vi "state machine 2.vi"() -> ()   [LabVIEW 2017]
uses:
  <vilib>/Platform/TimedLoop/XDataNode/timing_clust.ctl
  <vilib>/Platform/TimedLoop/XDataNode/nitl_modes.ctl
  <vilib>/Platform/TimedLoop/XDataNode/wakeup.ctl
  <vilib>/rvi/Emulation/niFpgaGetClockAttributes.vi
  <vilib>/rvi/Emulation/niFpgaSctlEmulationGetInTimedLoop.vi
  <vilib>/rvi/Emulation/niFpgaEmulationReportErrorSimple.vi
  <vilib>/rvi/Emulation/niFpgaProcessEmulError.vi
  <vilib>/rvi/Emulation/niFpgaCriticalErrorInLSC.vi
  <vilib>/rvi/interface/RandomDataEmulation/niFpgaRandomDataHandleErrors.vi
  <vilib>/rvi/eio/common/nirviEmuTemplateMethod_errors.vi
  <vilib>/Platform/TimedLoop/XDataNode/XDataNode.xnode
  <vilib>/rvi/DataTransferAndStorage/Container/XNode/niFpgaContainer.xnode
  <vilib>/rvi/interface/RandomDataEmulation/nirviRandomDataFpgaReadWriteTemplate.vi
  <vilib>/eio/EIONode/EIONode.xnode
  <vilib>/Platform/TimedLoop/XDataNode/XDNodeRunTimeDep.lvlib
panel:
  out "real-time port D monitor":bool[](array[boolean])
  out "real-time port C monitor":bool[](array[boolean])
  out "real-time port B monitor":bool[](array[boolean])
  out "real-time port A monitor":bool[](array[boolean])
  in  "stop":bool
  out "reset LED":bool
  out "run LED":bool
  in  "Reset":bool
  out "load LED":bool
  out "idle LED":bool
  in  "Run":bool
  in  "Load":bool
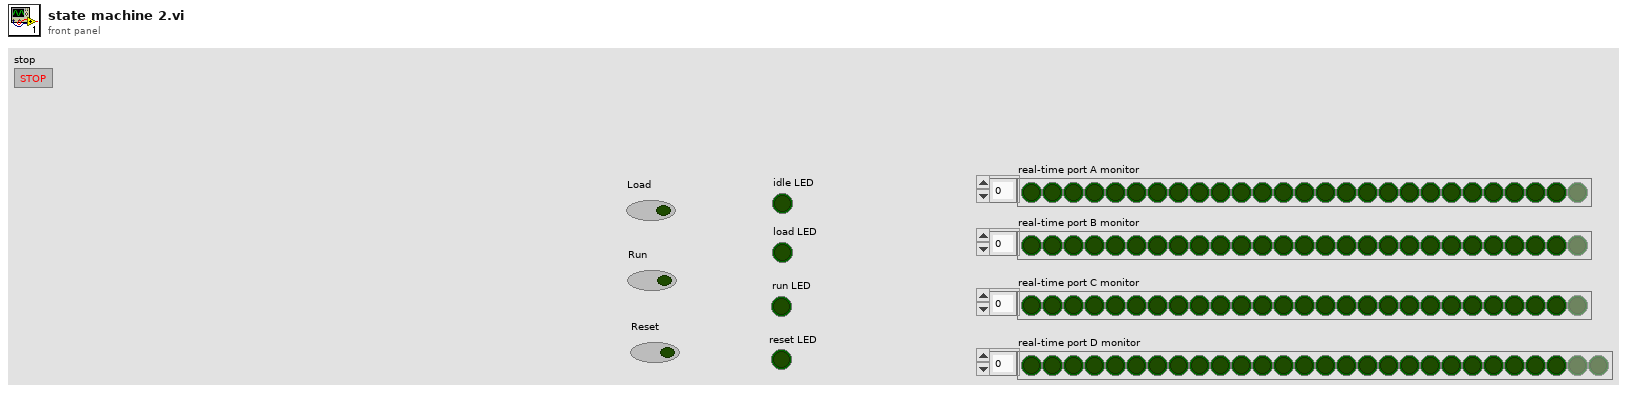
[diagram p1: front panel]
types:
  T1 = typedef "XDNodeRunTimeDep.lvlib/timing_clust.ctl" = cluster{"Expected End [f-1]":u64, "Actual End [f-1]":u64, "Finished Late? [f-1]":bool, "Expected End [i-1]":u64, "Actual End [i-1]":u64, "Finished Late? [i-1]":bool, "Expected Start [i]":u64, "Actual Start [i]":u64, "Expected Start [f]":u64, "Actual Start [f]":u64, "Source Name":string, "Structure Name":string, "Period":i64, "Deadline":i64, "Offset":i64, "Start":i64, "Priority":i32, "Timeout":i32, "Mode":T2, "Wakeup Reason":T3, "Error":errorcluster, "Source Type":string, "Secondary Source Type":string, "Global End Time":u64, "Global Start Time":u64, "Frame Duration":u64, "Iteration Duration":u64, "Assigned CPU":i32, "I/O Scan Engine Mode":u32}
  T2 = typedef "XDNodeRunTimeDep.lvlib/nitl_modes.ctl" = enum32{"No Change", "Process missed periods, maintain original phase", "Discard missed periods, maintain original phase", "Process missed periods, ignore original phase", "Discard missed periods, ignore original phase"}
  T3 = typedef "XDNodeRunTimeDep.lvlib/wakeup.ctl" = enum32{"Normal", "Aborted", "Asynchronous wakeup", "Timing source error", "Timed loop error", "Timeout"}
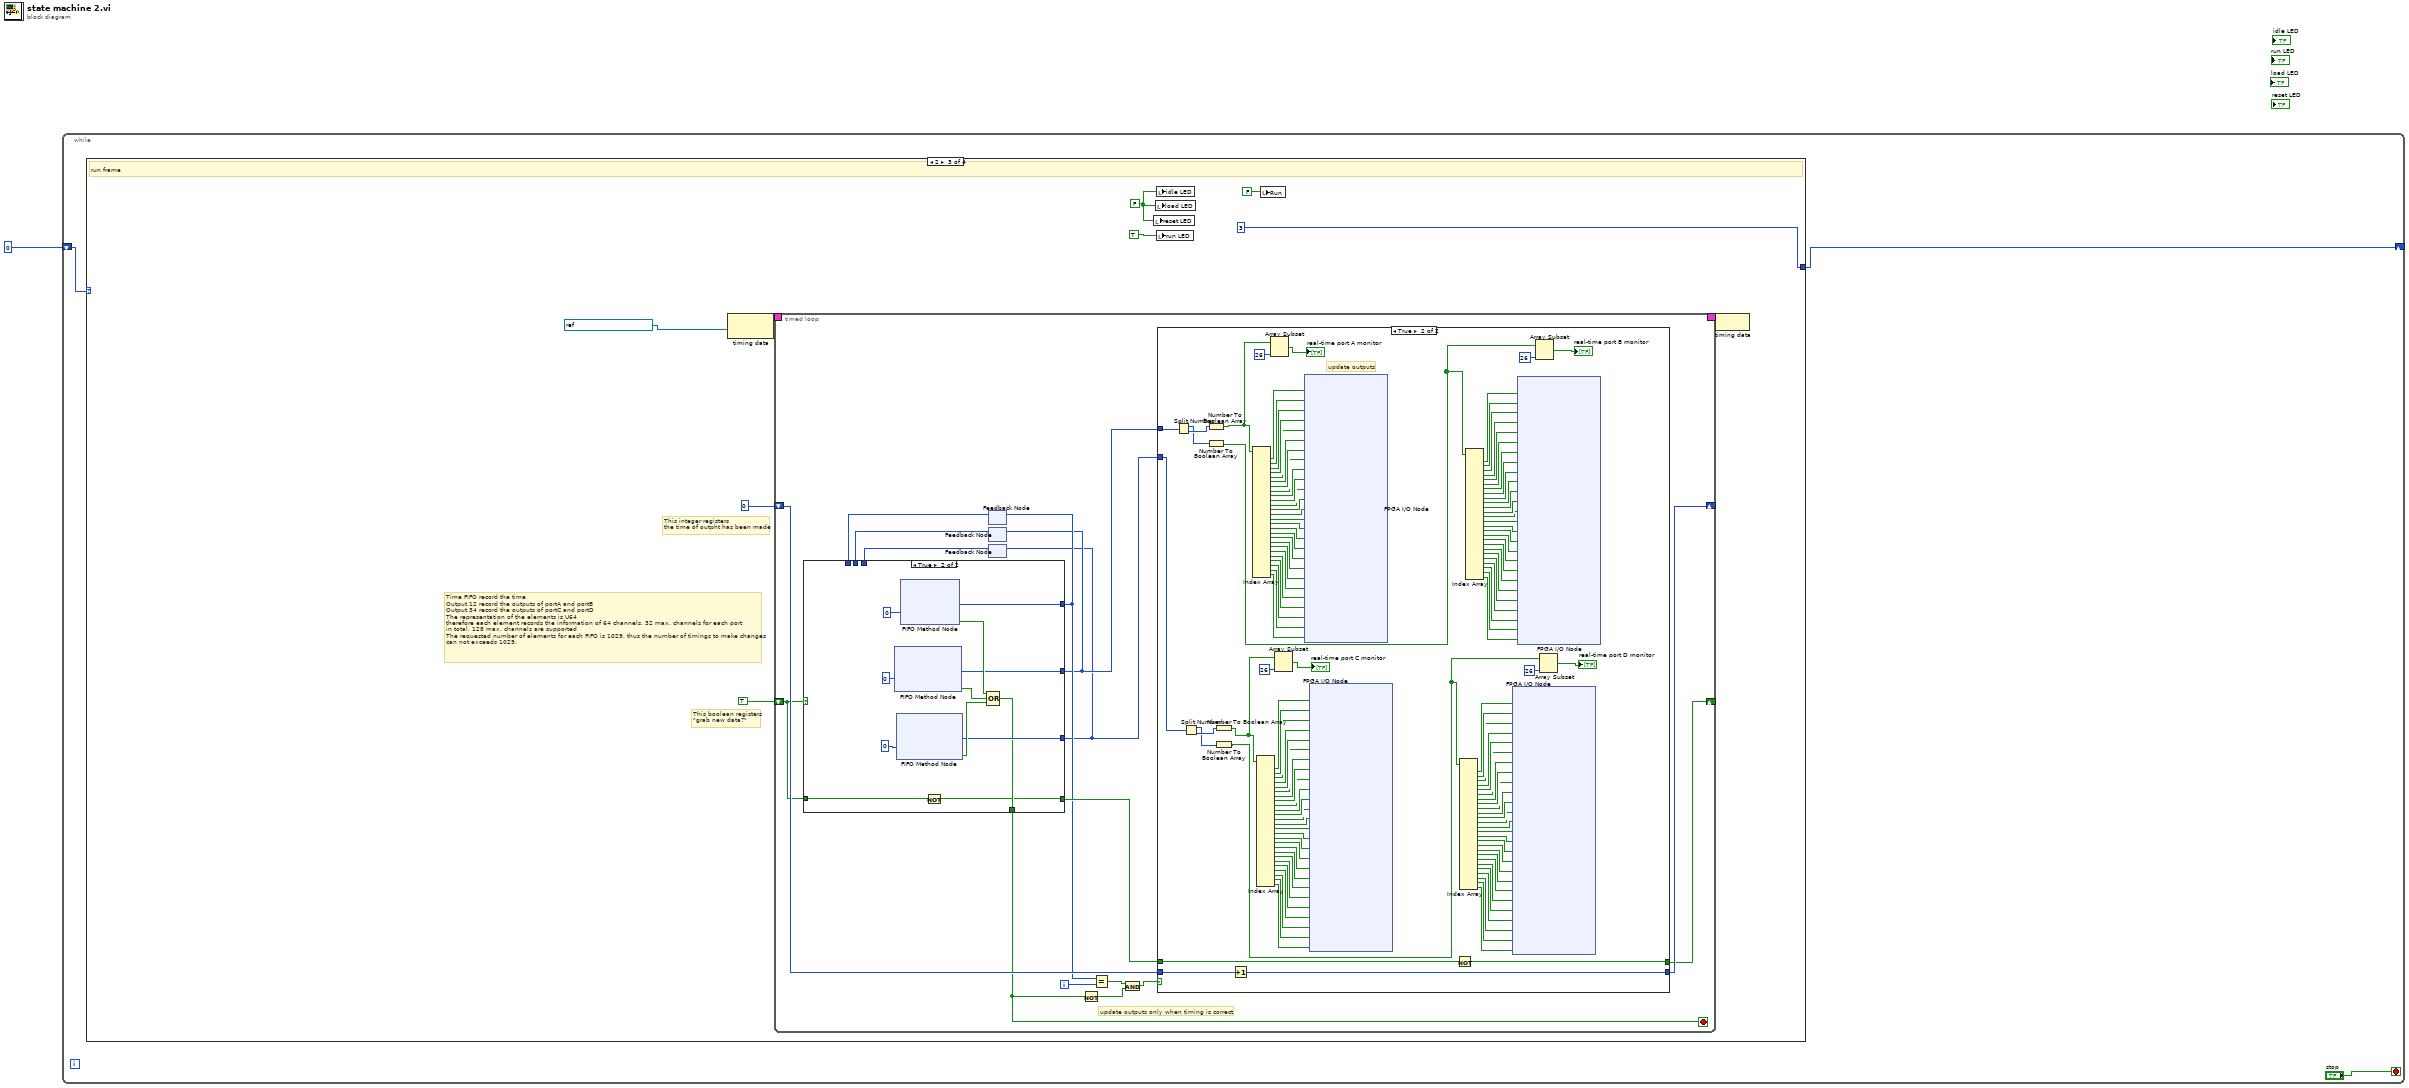
[diagram p0: block diagram]
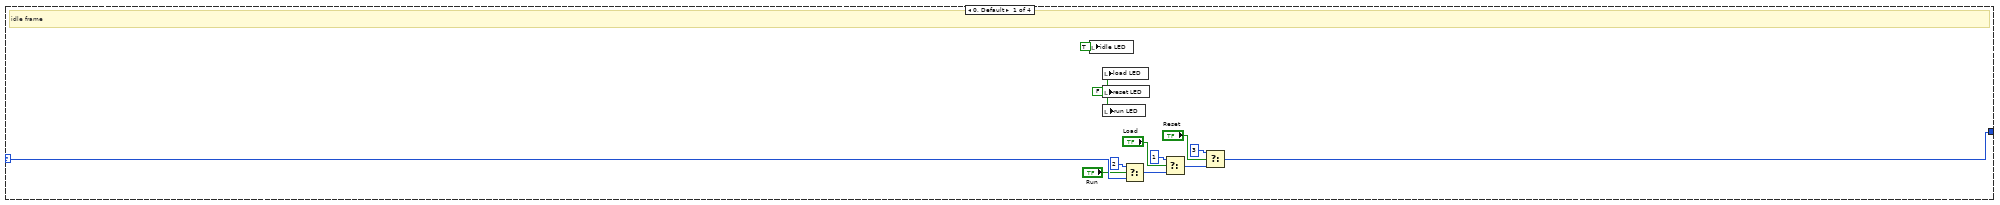
[diagram p2: hidden frame]
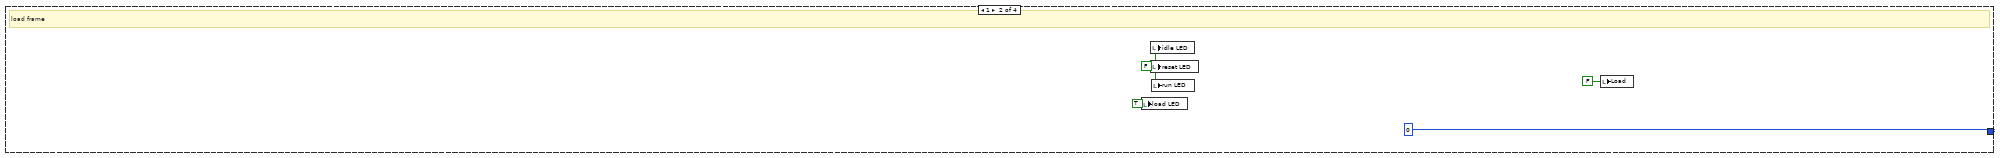
[diagram p3: hidden frame]
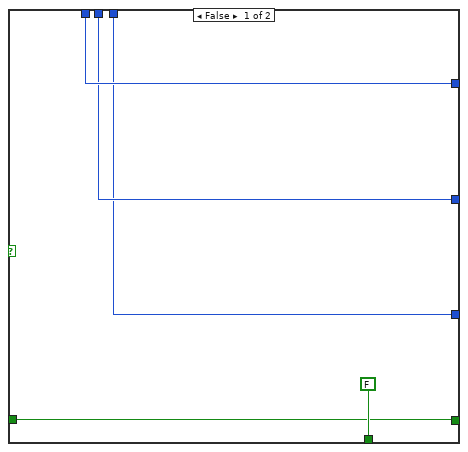
[diagram p4: hidden frame]
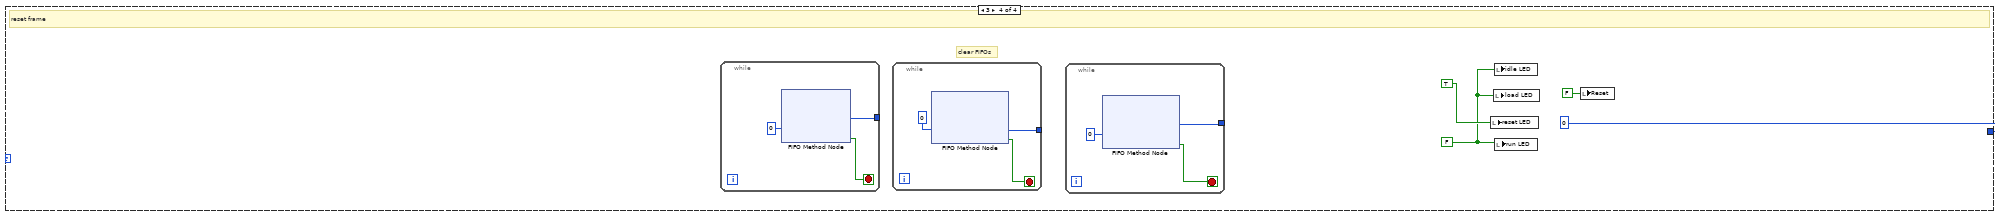
[diagram p6: hidden frame]
diagram:
  n1 = while {
    shift-right: [w3] -> _
    shift-left: i16 0 -> [w4]
    stop <- "stop" stop-if-true
    n2 = case shown="2" w4 {
      selector: w4 -> [w14 _ _ _]
      tunnel: [w7 i16 0 i16 3 i16 0] -> w3
      frame 0, Default {
        w15 = FALSE ("run")
        # "idle frame"
        n3 = local write "idle LED"(TRUE ("run")) -> ()
        n4 = local write "load LED"(w15) -> ()
        n5 = local write "reset LED"(w15) -> ()
        n6 = local write "run LED"(w15) -> ()
        n7 = Select(t=i16 2, s="Run", f=w14) -> (s? t:f=w11:i16)
        n8 = Select(t=i16 1, s="Load", f=w11) -> (s? t:f=w9:i16)
        n9 = Select(t=i16 3, s="Reset", f=w9) -> (s? t:f=w7:i16)
      }
      frame 1 {
        w20 = FALSE ("run")
        # "load frame"
        n10 = local write "load LED"(TRUE ("load")) -> ()
        n11 = local write "idle LED"(w20) -> ()
        n12 = local write "reset LED"(w20) -> ()
        n13 = local write "run LED"(w20) -> ()
        n14 = local write "Load"(FALSE) -> ()
      }
      frame 2 {
        w28 = FALSE ("run")
        # "This integer registers \nthe time of outpht has been made"
        # "This boolean registers\n\"grab new data?\""
        # "Time FIFO record the time\nOutput 12 record the outputs of portA and portB\nOutput 34 record the outputs of portC and portD\nThe representation of the elements is U64\ntherefore each element records the information of 64 channels, 32 max. channels for each port\nin total, 128 max. channels are supported\nThe requested number of elements for each FIFO is 1029, thus the number of timings to make changes \ncan not exceeds 1029."
        # "run frame"
        n15 = node-c288(refnum<k21> "40 MHz Onboard Clock" ("Source Name")) -> (w26:T1)
        n16 = timed-loop {
          timing: w26 -> [_]
          timing-out: [_] -> w25
          shift-right: [w43] -> _
          shift-left: i16 0 -> [w44]
          shift-right: [w37] -> _
          shift-left: TRUE ("Boolean") -> [w36]
          i -> [w45]
          stop <- w40 stop-if-true
          # "update outputs only when timing is correct"
          n17 = feedback #1() -> (w32:u64)  [unwired: 1 in]
          n18 = feedback #2() -> (w31:u64)  [unwired: 1 in]
          n19 = feedback #3() -> (w30:u64)  [unwired: 1 in]
          n20 = case shown="True" w36 {
            tunnel: [w47 w56] -> w34
            tunnel: [w46 w55] -> w33
            tunnel: [w48 w54] -> w35
            tunnel: [FALSE w53] -> w40
            tunnel: w36 -> [w49 w52]
            tunnel: [w49 w51] -> w38
            tunnel: w32 -> [w48 _]
            tunnel: w31 -> [w47 _]
            tunnel: w30 -> [w46 _]
            frame False {
            }
            frame True {
              n21 = xnode ("FIFO Method Node")("Timeout"=0) -> ("Element"=w56:u64, "Timed Out?"=w57:bool)  [unwired: 1 in, 1 out]
              n22 = xnode ("FIFO Method Node")("Timeout"=0) -> ("Element"=w55:u64, "Timed Out?"=w58:bool)  [unwired: 1 in, 1 out]
              n23 = xnode ("FIFO Method Node")("Timeout"=0) -> ("Element"=w54:u64, "Timed Out?"=w62:bool)  [unwired: 1 in, 1 out]
              n24 = Not(x=w52) -> (.not. x?=w51:bool)
              n25 = Compound Arithmetic op=OR(w62, w57, w58) -> (w53:bool)
            }
          }
          n26 = feedback-in #1(w35) -> ()
          n27 = feedback-in #2(w34) -> ()
          n28 = feedback-in #3(w33) -> ()
          n29 = Not(x=w40) -> (.not. x?=w39:bool)
          n30 = Equal?(x=w35, y=w45) -> (x = y?=w41:bool)
          n31 = And(x=w41, y=w39) -> (x .and. y?=w42:bool)
          n32 = case shown="True" w42 {
            tunnel: w34 -> [_ w134]
            tunnel: w33 -> [_ w67]
            tunnel: w44 -> [w64 w190]
            tunnel: [w64 w189] -> w43
            tunnel: w38 -> [w63 w75]
            tunnel: [w63 w74] -> w37
            frame False {
            }
            frame True {
              # "update outputs"
              n33 = Split Number(x=w134) -> (hi(x)=w71:u32, lo(x)=w73:u32)
              n34 = Split Number(x=w67) -> (hi(x)=w68:u32, lo(x)=w69:u32)
              n35 = Number To Boolean Array(number=w73) -> (Boolean array=w72:bool[])
              n36 = Number To Boolean Array(number=w71) -> (Boolean array=w70:bool[])
              n37 = Number To Boolean Array(number=w69) -> (Boolean array=w65:bool[])
              n38 = Number To Boolean Array(number=w68) -> (Boolean array=w66:bool[])
              n39 = Increment(x=w190) -> (x+1=w189:i16)
              n40 = Index Array(array=w72) -> (element #1=w188:bool, element #2=w187:bool, element #3=w186:bool, element #4=w185:bool, element #5=w184:bool, element #6=w183:bool, element #7=w182:bool, element #8=w181:bool, element #9=w180:bool, element #10=w179:bool, element #11=w178:bool, element #12=w177:bool, element #13=w176:bool, element #14=w175:bool, element #15=w174:bool, element #16=w173:bool, element #17=w172:bool, element #18=w171:bool, element #19=w170:bool, element #20=w169:bool, element #21=w168:bool, element #22=w167:bool, element #23=w166:bool, element #24=w165:bool, element #25=w164:bool, element #26=w103:bool)  [unwired: 26 in]
              n41 = Index Array(array=w65) -> (element #1=w133:bool, element #2=w127:bool, element #3=w126:bool, element #4=w125:bool, element #5=w124:bool, element #6=w123:bool, element #7=w122:bool, element #8=w121:bool, element #9=w120:bool, element #10=w119:bool, element #11=w118:bool, element #12=w117:bool, element #13=w116:bool, element #14=w115:bool, element #15=w114:bool, element #16=w113:bool, element #17=w112:bool, element #18=w111:bool, element #19=w110:bool, element #20=w109:bool, element #21=w108:bool, element #22=w107:bool, element #23=w106:bool, element #24=w105:bool, element #25=w104:bool, element #26=w101:bool)  [unwired: 26 in]
              n42 = Array Subset(array=w72, length=26) -> (→"real-time port A monitor":bool[])  [unwired: 1 in]
              n43 = Array Subset(array=w65, length=26) -> (→"real-time port C monitor":bool[])  [unwired: 1 in]
              n44 = xnode "FPGA I/O Node"("Connector0/DIO0"=w188, "Connector0/DIO1"=w187, "Connector0/DIO2"=w186, "Connector0/DIO3"=w185, "Connector0/DIO4"=w184, "Connector0/DIO5"=w183, "Connector0/DIO6"=w182, "Connector0/DIO7"=w181, "Connector0/DIO8"=w180, "Connector0/DIO9"=w179, "Connector0/DIO10"=w178, "Connector0/DIO11"=w177, "Connector0/DIO12"=w176, "Connector0/DIO13"=w175, "Connector0/DIO14"=w174, "Connector0/DIO15"=w173, "Connector0/DIO16"=w172, "Connector0/DIO17"=w171, "Connector0/DIO18"=w170, "Connector0/DIO19"=w169, "Connector0/DIO20"=w168, "Connector0/DIO21"=w167, "Connector0/DIO22"=w166, "Connector0/DIO23"=w165, "Connector0/DIO24"=w164, "Connector0/DIO25"=w103) -> ()  [unwired: 26 in, 26 out]
              n45 = xnode "FPGA I/O Node"("Connector2/DIO0"=w133, "Connector2/DIO1"=w127, "Connector2/DIO2"=w126, "Connector2/DIO3"=w125, "Connector2/DIO4"=w124, "Connector2/DIO5"=w123, "Connector2/DIO6"=w122, "Connector2/DIO7"=w121, "Connector2/DIO8"=w120, "Connector2/DIO9"=w119, "Connector2/DIO10"=w118, "Connector2/DIO11"=w117, "Connector2/DIO12"=w116, "Connector2/DIO13"=w115, "Connector2/DIO14"=w114, "Connector2/DIO15"=w113, "Connector2/DIO16"=w112, "Connector2/DIO17"=w111, "Connector2/DIO18"=w110, "Connector2/DIO19"=w109, "Connector2/DIO20"=w108, "Connector2/DIO21"=w107, "Connector2/DIO22"=w106, "Connector2/DIO23"=w105, "Connector2/DIO24"=w104, "Connector2/DIO25"=w101) -> ()  [unwired: 26 in, 26 out]
              n46 = Not(x=w75) -> (.not. x?=w74:bool)
              n47 = Index Array(array=w66) -> (element #1=w132:bool, element #2=w100:bool, element #3=w99:bool, element #4=w98:bool, element #5=w97:bool, element #6=w96:bool, element #7=w95:bool, element #8=w94:bool, element #9=w93:bool, element #10=w92:bool, element #11=w91:bool, element #12=w90:bool, element #13=w89:bool, element #14=w88:bool, element #15=w87:bool, element #16=w86:bool, element #17=w85:bool, element #18=w84:bool, element #19=w83:bool, element #20=w82:bool, element #21=w81:bool, element #22=w80:bool, element #23=w79:bool, element #24=w78:bool, element #25=w77:bool, element #26=w76:bool)  [unwired: 26 in]
              n48 = Index Array(array=w70) -> (element #1=w163:bool, element #2=w162:bool, element #3=w161:bool, element #4=w160:bool, element #5=w159:bool, element #6=w158:bool, element #7=w157:bool, element #8=w156:bool, element #9=w155:bool, element #10=w154:bool, element #11=w153:bool, element #12=w152:bool, element #13=w151:bool, element #14=w150:bool, element #15=w149:bool, element #16=w148:bool, element #17=w147:bool, element #18=w146:bool, element #19=w145:bool, element #20=w144:bool, element #21=w143:bool, element #22=w142:bool, element #23=w141:bool, element #24=w140:bool, element #25=w139:bool, element #26=w102:bool)  [unwired: 26 in]
              n49 = xnode "FPGA I/O Node"("Connector3/DIO0"=w132, "Connector3/DIO1"=w100, "Connector3/DIO2"=w99, "Connector3/DIO3"=w98, "Connector3/DIO4"=w97, "Connector3/DIO5"=w96, "Connector3/DIO6"=w95, "Connector3/DIO7"=w94, "Connector3/DIO8"=w93, "Connector3/DIO9"=w92, "Connector3/DIO10"=w91, "Connector3/DIO11"=w90, "Connector3/DIO12"=w89, "Connector3/DIO13"=w88, "Connector3/DIO14"=w87, "Connector3/DIO15"=w86, "Connector3/DIO16"=w85, "Connector3/DIO17"=w84, "Connector3/DIO18"=w83, "Connector3/DIO19"=w82, "Connector3/DIO20"=w81, "Connector3/DIO21"=w80, "Connector3/DIO22"=w79, "Connector3/DIO23"=w78, "Connector3/DIO24"=w77, "Connector3/DIO25"=w76) -> ()  [unwired: 26 in, 26 out]
              n50 = xnode "FPGA I/O Node"("Connector1/DIO0"=w163, "Connector1/DIO1"=w162, "Connector1/DIO2"=w161, "Connector1/DIO3"=w160, "Connector1/DIO4"=w159, "Connector1/DIO5"=w158, "Connector1/DIO6"=w157, "Connector1/DIO7"=w156, "Connector1/DIO8"=w155, "Connector1/DIO9"=w154, "Connector1/DIO10"=w153, "Connector1/DIO11"=w152, "Connector1/DIO12"=w151, "Connector1/DIO13"=w150, "Connector1/DIO14"=w149, "Connector1/DIO15"=w148, "Connector1/DIO16"=w147, "Connector1/DIO17"=w146, "Connector1/DIO18"=w145, "Connector1/DIO19"=w144, "Connector1/DIO20"=w143, "Connector1/DIO21"=w142, "Connector1/DIO22"=w141, "Connector1/DIO23"=w140, "Connector1/DIO24"=w139, "Connector1/DIO25"=w102) -> ()  [unwired: 26 in, 26 out]
              n51 = Array Subset(array=w70, length=26) -> (→"real-time port B monitor":bool[])  [unwired: 1 in]
              n52 = Array Subset(array=w66, length=26) -> (→"real-time port D monitor":bool[])  [unwired: 1 in]
            }
          }
        }
        n53 = local write "reset LED"(w28) -> ()
        n54 = local write "load LED"(w28) -> ()
        n55 = local write "idle LED"(w28) -> ()
        n56 = local write "run LED"(TRUE ("run")) -> ()
        n57 = local write "Run"(FALSE) -> ()
        n58 = node-c288(w25) -> ()
      }
      frame 3 {
        w199 = FALSE ("run")
        # "clear FIFOs"
        # "reset frame"
        n59 = while {
          tunnel: [w209] -> _
          stop <- w207 stop-if-true
          n60 = xnode ("FIFO Method Node")("Timeout"=0) -> ("Element"=w209:u64, "Timed Out?"=w207:bool)  [unwired: 1 in, 1 out]
        }
        n61 = while {
          tunnel: [w204] -> _
          stop <- w205 stop-if-true
          n62 = xnode ("FIFO Method Node")("Timeout"=0) -> ("Element"=w204:u64, "Timed Out?"=w205:bool)  [unwired: 1 in, 1 out]
        }
        n63 = while {
          tunnel: [w201] -> _
          stop <- w202 stop-if-true
          n64 = xnode ("FIFO Method Node")("Timeout"=0) -> ("Element"=w201:u64, "Timed Out?"=w202:bool)  [unwired: 1 in, 1 out]
        }
        n65 = local write "reset LED"(TRUE ("run")) -> ()
        n66 = local write "load LED"(w199) -> ()
        n67 = local write "idle LED"(w199) -> ()
        n68 = local write "run LED"(w199) -> ()
        n69 = local write "Reset"(FALSE) -> ()
      }
    }
  }
